vi "niDTS BT INSTR RX Configure Hardware Parameters.vi"(8 "error in (no error)":errorcluster, 11 "niDTS BT INSTR RX in":refnum<class "niDTS BT INSTR RX.lvclass">) -> (0 "error out":errorcluster, 3 "niDTS BT INSTR RX out":refnum<class "niDTS BT INSTR RX.lvclass">)   [LabVIEW 2015, in "niDTS BT.lvlib" / "niDTS BT INSTR RX.lvclass"]
uses:
  niDTS BT INSTR RX.lvclass
  niDTS BT INSTR RX.lvclass/niDTS BT INSTR RX.ctl
  RiviInstDriver/niRfsgBT/Objects/niRfsgBt.lvclass
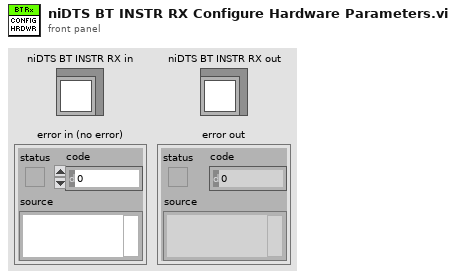
[diagram p1: front panel]
types:
  T1 = typedef "niRfsgBT.lvclass/niRfsgBT INC Handle.ctl" = refnum<data-value>
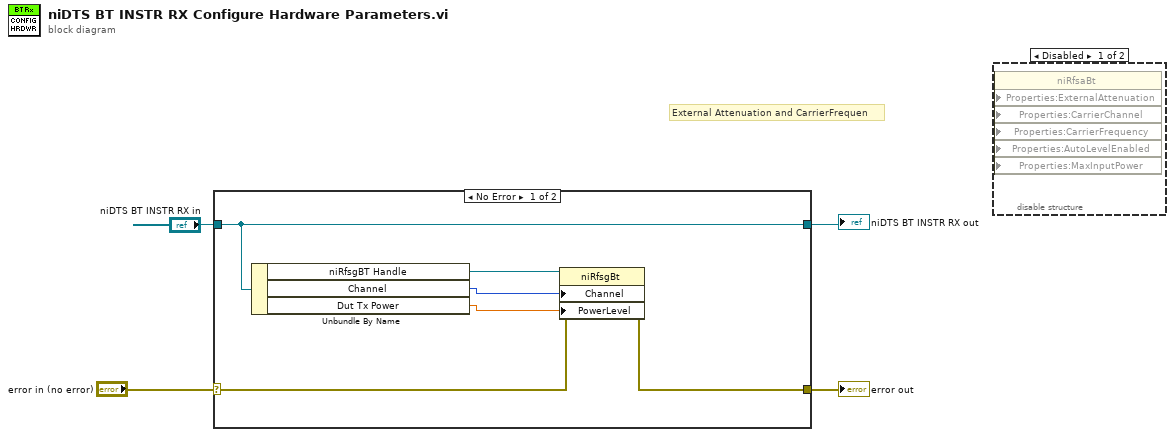
[diagram p0: block diagram]
diagram:
  # "External Attenuation and CarrierFrequen"
  n1 = case shown="No Error" "error in (no error)" {
    selector: "error in (no error)" -> [w10 w12]
    tunnel: [w9 w12] -> w3
    tunnel: [w6 w11] -> w1
    tunnel: "niDTS BT INSTR RX in" -> [w6 w11]
    frame No Error {
      n2 = Unbundle By Name(w6) -> ("niRfsgBT Handle"=w8:T1, "Channel"=w7:i32, "Dut Tx Power"=w5:dbl)
      n3 = property class="niRfsgBt"(reference=w8, error in=w10, "Channel"=w7, "PowerLevel"=w5) -> (error out=w9:errorcluster)  [unwired: 1 out]
    }
    frame Error {
    }
  }
  "error out" <- w3
  "niDTS BT INSTR RX out" <- w1
  n4 = disable-structure shown="Disabled" {
    frame Disabled {
      n5 = property class="niRfsaBt" props=["Properties:ExternalAttenuation", "Properties:CarrierChannel", "Properties:CarrierFrequency", "Properties:AutoLevelEnabled", "Properties:MaxInputPower"]() -> ()  [unwired: 7 in, 2 out]
    }
    frame Enabled {
    }
  }
